vi "Disable Modulationl.vi"(0 "VISA resource name":refnum<visa-resource-name>, 5 "Modulation":u32(ring) items=["Not Available", "Available"], 11 "error in (no error)":errorcluster) -> (4 "VISA resource name out":refnum<visa-resource-name>, 15 "error out":errorcluster)   [LabVIEW 2022 SP3, in "MagnaDC.lvlib"]
uses:
  MagnaDC.lvlib
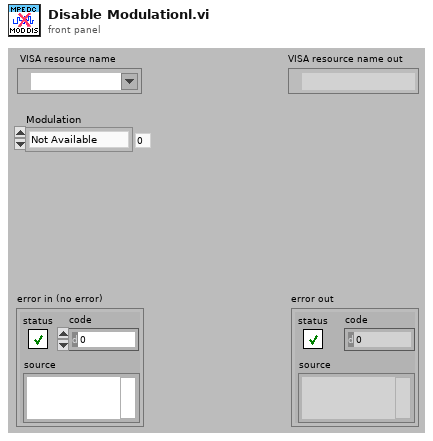
[diagram p1: front panel]
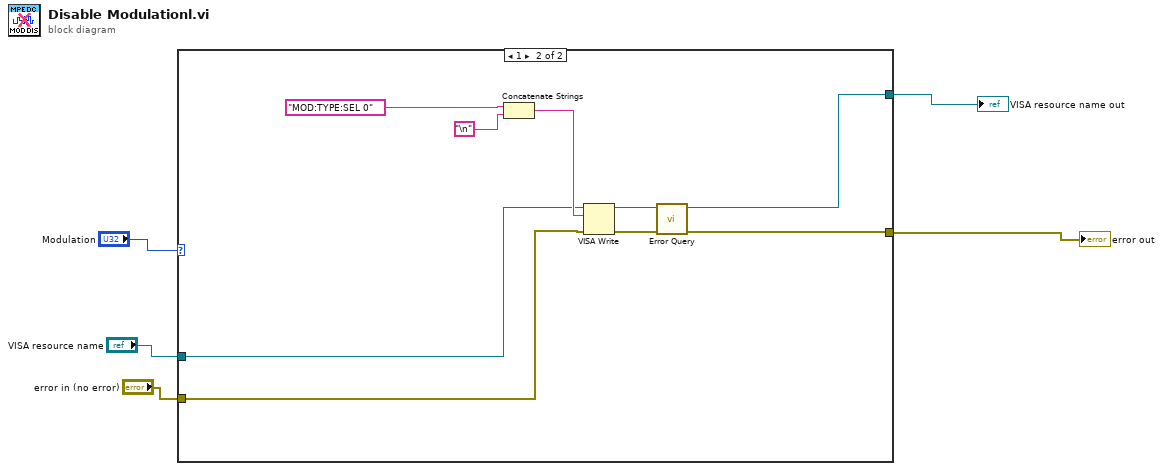
[diagram p0: block diagram]
diagram:
  n1 = case shown="1" "Modulation" {
    tunnel: "VISA resource name" -> [w6 w11]
    tunnel: "error in (no error)" -> [w7 w10]
    tunnel: [w6 w8] -> w1
    tunnel: [w7 w12] -> w2
    frame 0, Default {
    }
    frame 1 {
      n2 = Concatenate Strings("MOD:TYPE:SEL 0", "\n") -> (w13:string)
      n3 = VISA Write(VISA resource name=w11, write buffer=w13, error in (no error)=w10) -> (VISA resource name out=w16:refnum<visa-resource-name>, error out=w15:errorcluster)  [unwired: 1 out]
      n4 = call "Error Query.vi"("error in (no error)"=w15, "VISA resource name"=w16) -> ("error out"=w12:errorcluster, "VISA resource name out"=w8:refnum<visa-resource-name>)  [unwired: 6 in, 2 out]
    }
  }
  "error out" <- w2
  "VISA resource name out" <- w1
